vi "AB_Engine_RESTful_Validate_Template_Type.vi"(9 "source file names":string[](array[string]), 11 "RESTful VI routing template in":T1) -> (1 "template type vald":bool, 3 "source file index":i32)   [LabVIEW 2020]
uses:
  <vilib>/AppBuilder/AB_Classes/RESTful/AB_RESTful_RoutingTemplate.ctl
  <vilib>/AppBuilder/AB_Classes/RESTful/AB_RESTful_RoutingType.ctl
  <vilib>/AppBuilder/AB_Classes/RESTful/AB_RESTful_HTTPMethodType.ctl
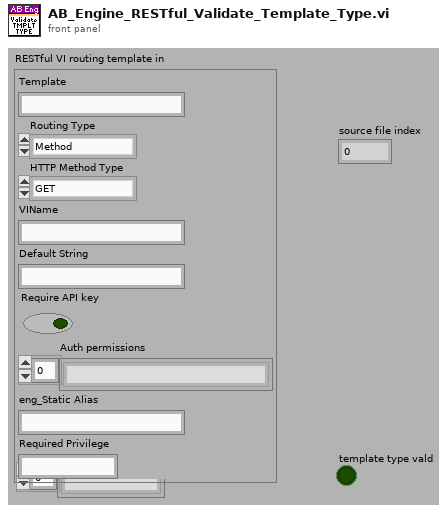
[diagram p1: front panel]
types:
  T1 = typedef "AB_RESTful_RoutingTemplate.ctl" = cluster{"Template":string, "Routing Type":T2, "HTTP Method Type":T3, "VIName":string, "Default String":string, "Require API key":bool, "Auth permissions":string[], "eng_Static Alias":string, "Required Privilege":string}
  T2 = typedef "AB_RESTful_RoutingType.ctl" = enum32{"Method", "Static"}
  T3 = typedef "AB_RESTful_HTTPMethodType.ctl" = enum32{"GET", "POST", "PUT", "DELETE"}
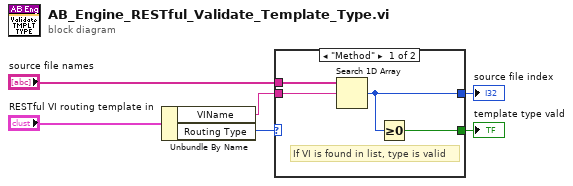
[diagram p0: block diagram]
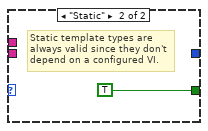
[diagram p2: hidden frame]
diagram:
  n1 = Unbundle By Name("RESTful VI routing template in") -> ("VIName"=w2:string, "Routing Type"=w1:T2)
  n2 = case shown="\"Method\"" w1 {
    tunnel: [w10 _] -> w4
    tunnel: "source file names" -> [w9 _]
    tunnel: w2 -> [w8 _]
    tunnel: [w7 TRUE] -> w5
    frame "Method" {
      # "If VI is found in list, type is valid"
      n3 = Search 1D Array(1D array=w9, element=w8) -> (index of element=w10:i32)  [unwired: 1 in]
      n4 = Greater Or Equal To 0?(x=w10) -> (x >= 0?=w7:bool)
    }
    frame "Static" {
      # "Static template types are always valid since they don't depend on a configured VI."
    }
  }
  "template type vald" <- w5
  "source file index" <- w4
